vi "Save VI.vi"(4 "Control[] (Empty: all)":refnum<vi>[](array[refnum]), 6 "Section Name (\"Settings\")":string="Settings", 8 "error in (no error)":errorcluster, 9 "Path":path, 10 "VI Reference In (Caller)":refnum<vi>, 11 "Save Restore Settings in":refnum<class "Save Restore Settings.lvclass">) -> (0 "error out":errorcluster, 2 "VI Reference Out":refnum<vi>, 3 "Save Restore Settings out":refnum<class "Save Restore Settings.lvclass">)   [LabVIEW 2016, in "Save Restore Settings.lvclass"]
doc: "Saves a settings file for the specified VI, including panel bounds, splitter bar positions, listbox column widths, and graph/chart plots. The settings are saved in an ini file at the specified path. The <B>Save Restore Settings in</B> class may be supplied with a child class to customize what properties are saved. \nPlease see the description for <B>MGI Save Restore Settings.lvclass:Load VI.vi</B> for more details\n\nAuthored by Shawn Walpole\nsupport@mooregoodideas.com\nwww.mooregoodideas.com\n\nCopyright (c) 2010, Moore Good Ideas, Inc.\n\nAll rights reserved.\n\nRedistribution and use in source and binary forms, with or without modification, are permitted provided that the following conditions are met:\n\n * Redistributions of source code must retain the above copyright notice, this list of conditions and the following disclaimer.\n * Redistributions in binary form must reproduce the above copyright notice, this list of conditions and the following disclaimer in the documentation and/or other materials provided with the distribution.\n * Neither the name of Moore Good Ideas, Inc. nor the names of its contributors may be used to endorse or promote products derived from this software without specific prior written permission.\n\nTHIS SOFTWARE IS PROVIDED BY THE COPYRIGHT HOLDERS AND CONTRIBUTORS \"AS IS\" AND ANY EXPRESS OR IMPLIED WARRANTIES, INCLUDING, BUT NOT LIMITED TO, THE IMPLIED WARRANTIES OF MERCHANTABILITY AND FITNESS FOR A PARTICULAR PURPOSE ARE DISCLAIMED. IN NO EVENT SHALL THE COPYRIGHT OWNER OR CONTRIBUTORS BE LIABLE FOR ANY DIRECT, INDIRECT, INCIDENTAL, SPECIAL, EXEMPLARY, OR CONSEQUENTIAL DAMAGES (INCLUDING, BUT NOT LIMITED TO, PROCUREMENT OF SUBSTITUTE GOODS OR SERVICES; LOSS OF USE, DATA, OR PROFITS; OR BUSINESS INTERRUPTION) HOWEVER CAUSED AND ON ANY THEORY OF LIABILITY, WHETHER IN CONTRACT, STRICT LIABILITY, OR TORT (INCLUDING NEGLIGENCE OR OTHERWISE) ARISING IN ANY WAY OUT OF THE USE OF THIS SOFTWARE, EVEN IF ADVISED OF THE POSSIBILITY OF SUCH DAMAGE."
uses:
  <userlib>/_MGI/Application Control/MGI Save Restore Settings/Save Restore Settings.lvclass
  <userlib>/_MGI/Application Control/MGI VI Reference/MGI Caller's VI Reference.vi
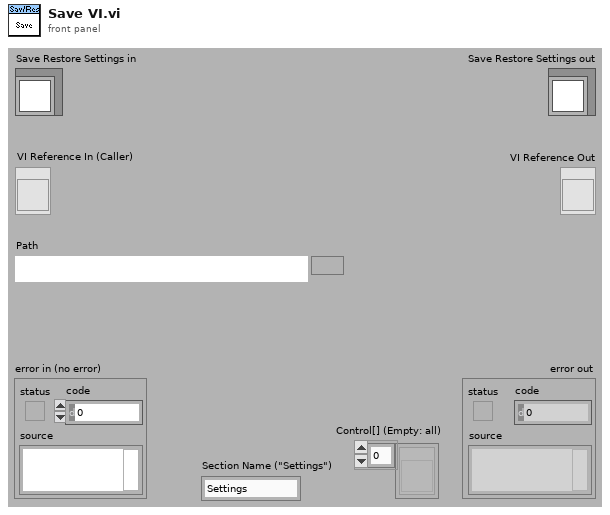
[diagram p1: front panel]
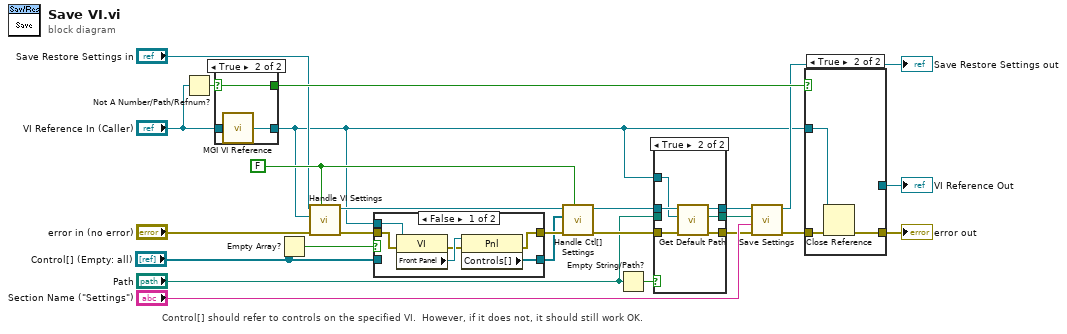
[diagram p0: block diagram]
diagram:
  w16 = FALSE ("Write? (F:Read)")
  # "Control[] should refer to controls on the specified VI.  However, if it does not, it should still work OK."
  n1 = Not A Number/Path/Refnum?(number/path/refnum="VI Reference In (Caller)") -> (NaN/Path/Refnum?=w25:bool)
  n2 = case shown="True" w25 {
    selector: w25 -> [_ w27]
    tunnel: [w26 w28] -> w3
    tunnel: "VI Reference In (Caller)" -> [w26 _]
    tunnel: [_ w27] -> w22
    frame False {
    }
    frame True {
      n3 = call-poly <userlib>:"MGI VI Reference.vi"() -> ("Caller's VI Reference"=w28:refnum<vi>)  [unwired: 1 in]
    }
  }
  n4 = Empty Array?(array="Control[] (Empty: all)") -> (empty?=w2:bool)
  n5 = call-dynamic "Handle VI Settings.vi"("Write VI? (F:Read)"=w16, "error in (no error)"="error in (no error)", "VI Refnum"=w3, "Save Restore Settings in"="Save Restore Settings in") -> ("error out"=w6:errorcluster, "Save Restore Settings out"=w23:refnum<class "Save Restore Settings.lvclass">)  [unwired: 6 in]
  n6 = case shown="False" w2 {
    tunnel: w6 -> [w32 w35]
    tunnel: [w31 w35] -> w5
    tunnel: [w30 w36] -> w4
    tunnel: w3 -> [w29 _]
    tunnel: "Control[] (Empty: all)" -> [_ w36]
    frame False {
      n7 = property class="VI"(reference=w29, error in=w32) -> (error out=w33:errorcluster, "Front Panel"=w34:refnum<vi>)  [unwired: 1 out]
      n8 = property class="Pnl"(reference=w34, error in=w33) -> (error out=w31:errorcluster, "Controls[]"=w30:refnum<vi>[])  [unwired: 1 out]
    }
    frame True {
    }
  }
  n9 = call-dynamic "Handle Ctl[] Settings.vi"("Write Ctl? (F:Read)"=w16, "error in (no error)"=w5, "Controls[]"=w4, "Save Restore Settings in"=w23) -> ("error out"=w13:errorcluster, "Save Restore Settings out"=w9:refnum<class "Save Restore Settings.lvclass">)  [unwired: 6 in]
  n10 = Empty String/Path?(string/path="Path") -> (empty?=w15:bool)
  n11 = case shown="True" w15 {
    tunnel: w13 -> [w37 w45]
    tunnel: [w37 w44] -> w11
    tunnel: "Path" -> [w39 _]
    tunnel: w9 -> [w38 w43]
    tunnel: [w38 w42] -> w8
    tunnel: [w39 w41] -> w12
    tunnel: w3 -> [_ w40]
    frame False {
    }
    frame True {
      n12 = call-dynamic "Get Default Path.vi"("error in (no error)"=w45, "VI Refnum"=w40, "Save Restore Settings in"=w43) -> ("error out"=w44:errorcluster, "Default Path"=w41:path, "Save Restore Settings out"=w42:refnum<class "Save Restore Settings.lvclass">)  [unwired: 6 in]
    }
  }
  n13 = call-dynamic "Save Settings.vi"("error in (no error)"=w11, "Section"="Section Name (\"Settings\")", "Path"=w12, "Save Restore Settings in"=w8) -> ("error out"=w18:errorcluster, "Save Restore Settings out"=→"Save Restore Settings out":refnum<class "Save Restore Settings.lvclass">)  [unwired: 6 in]
  n14 = case shown="True" w22 {
    tunnel: w18 -> [w47 w50]
    tunnel: [w47 w48] -> w21
    tunnel: w3 -> [w46 w49]
    tunnel: [w46 _] -> w20
    frame False {
    }
    frame True {
      n15 = Close Reference(reference=w49, error in (no error)=w50) -> (error out=w48:errorcluster)
    }
  }
  "error out" <- w21
  "VI Reference Out" <- w20
